vi "Write directory.vi"(8 "error in (no error)":errorcluster, 10 "directory":path, 11 "Log File in":refnum<class "CM_Log File.lvclass">) -> (0 "error out":errorcluster, 3 "Log File out":refnum<class "CM_Log File.lvclass">)   [LabVIEW 2018, in "CM_Log File.lvclass"]
uses:
  CM_Log File.lvclass
  CM_Log File.lvclass/CM_Log File.ctl
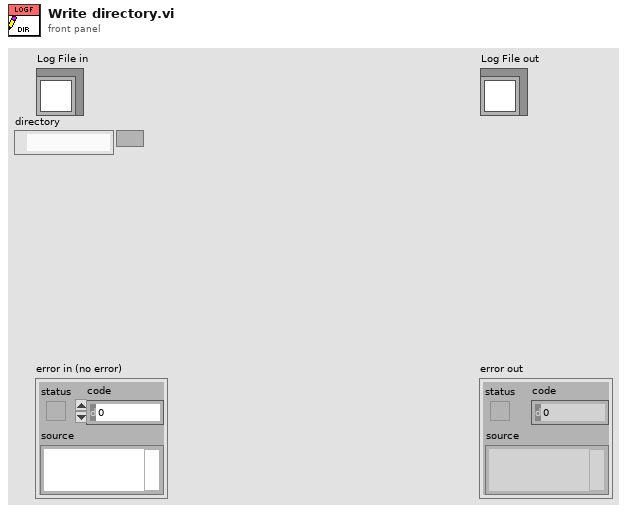
[diagram p1: front panel]
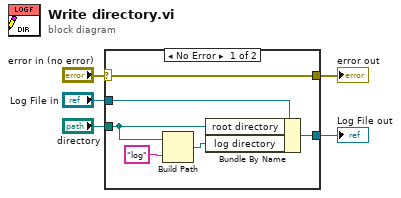
[diagram p0: block diagram]
diagram:
  n1 = case shown="No Error" "error in (no error)" {
    selector: "error in (no error)" -> [w9 w12]
    tunnel: [w9 w12] -> w4
    tunnel: [w10 w13] -> w2
    tunnel: "Log File in" -> [w11 w13]
    tunnel: "directory" -> [w8 _]
    frame No Error {
      n2 = Build Path(base path=w8, name or relative path="log") -> (appended path=w6:path)
      n3 = Bundle By Name(cluster=w11, "root directory"=w8, "log directory"=w6) -> (w10:refnum<class "CM_Log File.lvclass">)
    }
    frame Error {
    }
  }
  "error out" <- w4
  "Log File out" <- w2
